vi "XXPathPlanner_Path_RePlan_Worker2.vi"(4 "StartingPoseTranslation":T11 {"Y" format="%14.3f"; "X" format="%14.3f"}, 5 "in PathPlannerPath":T1={"Reversed"=FALSE, "RotationTargets"=[], "ConstraintZones"=[], "EventMarkers"=[], "GlobalConstraints"={"MaxVelocityMps;"=0.0, "MaxAccelerationMpsSq;"=0.0, "MaxAngularVelRadPsEc;"=0.0, "MaxAngularAccRadPSecSq"=0.0, "Exists"=FALSE, "Unlimited"=FALSE, "NominalVoltageVolts"=12.0}, "GoalEndState"={"VelocityMPS"=0.0, "Rotation"={"VALUE"=0.0, "COS"=0.0, "SIN"=0.0}}, "AllPoints"=[], "Name"="", "Waypoints"=[], "PointTowardsZones"=[], "IdealStartingState"={"VelocityMPS"=0.0, "Rotation"={"VALUE"=0.0, "COS"=0.0, "SIN"=0.0}}, "IsChoreoPath"=FALSE, "PreventFlipping"=FALSE} {"IdealStartingState"."Rotation"."SIN" format="%13.4f"; "IdealStartingState"."Rotation"."COS" format="%13.4f"; "IdealStartingState"."Rotation"."VALUE" format="%13.4f"; "PointTowardsZones"."TargetPosition"."Y" format="%14.3f"; "PointTowardsZones"."TargetPosition"."X" format="%14.3f"; "PointTowardsZones"."RotationOffset"."SIN" format="%13.4f"; "PointTowardsZones"."RotationOffset"."COS" format="%13.4f"; "PointTowardsZones"."RotationOffset"."VALUE" format="%13.4f"; "Waypoints"."nextControl"."Y" format="%14.3f"; "Waypoints"."nextControl"."X" format="%14.3f"; "Waypoints"."anchor"."Y" format="%14.3f"; "Waypoints"."anchor"."X" format="%14.3f"; "Waypoints"."prevControl"."Y" format="%14.3f"; "Waypoints"."prevControl"."X" format="%14.3f"; "AllPoints"."RotationTarget"."rotation"."SIN" format="%13.4f"; "AllPoints"."RotationTarget"."rotation"."COS" format="%13.4f"; "AllPoints"."RotationTarget"."rotation"."VALUE" format="%13.4f"; "AllPoints"."Position"."Y" format="%14.3f"; "AllPoints"."Position"."X" format="%14.3f"; "GoalEndState"."Rotation"."SIN" format="%13.4f"; "GoalEndState"."Rotation"."COS" format="%13.4f"; "GoalEndState"."Rotation"."VALUE" format="%13.4f"; "RotationTargets"."rotation"."SIN" format="%13.4f"; "RotationTargets"."rotation"."COS" format="%13.4f"; "RotationTargets"."rotation"."VALUE" format="%13.4f"}) -> (2 "Error":bool, 3 "Replanned Path":T1={"Reversed"=FALSE, "RotationTargets"=[], "ConstraintZones"=[], "EventMarkers"=[], "GlobalConstraints"={"MaxVelocityMps;"=0.0, "MaxAccelerationMpsSq;"=0.0, "MaxAngularVelRadPsEc;"=0.0, "MaxAngularAccRadPSecSq"=0.0, "Exists"=FALSE, "Unlimited"=FALSE, "NominalVoltageVolts"=12.0}, "GoalEndState"={"VelocityMPS"=0.0, "Rotation"={"VALUE"=0.0, "COS"=0.0, "SIN"=0.0}}, "AllPoints"=[], "Name"="", "Waypoints"=[], "PointTowardsZones"=[], "IdealStartingState"={"VelocityMPS"=0.0, "Rotation"={"VALUE"=0.0, "COS"=0.0, "SIN"=0.0}}, "IsChoreoPath"=FALSE, "PreventFlipping"=FALSE} {"IdealStartingState"."Rotation"."SIN" format="%13.4f"; "IdealStartingState"."Rotation"."COS" format="%13.4f"; "IdealStartingState"."Rotation"."VALUE" format="%13.4f"; "PointTowardsZones"."TargetPosition"."Y" format="%14.3f"; "PointTowardsZones"."TargetPosition"."X" format="%14.3f"; "PointTowardsZones"."RotationOffset"."SIN" format="%13.4f"; "PointTowardsZones"."RotationOffset"."COS" format="%13.4f"; "PointTowardsZones"."RotationOffset"."VALUE" format="%13.4f"; "Waypoints"."nextControl"."Y" format="%14.3f"; "Waypoints"."nextControl"."X" format="%14.3f"; "Waypoints"."anchor"."Y" format="%14.3f"; "Waypoints"."anchor"."X" format="%14.3f"; "Waypoints"."prevControl"."Y" format="%14.3f"; "Waypoints"."prevControl"."X" format="%14.3f"; "AllPoints"."RotationTarget"."rotation"."SIN" format="%13.4f"; "AllPoints"."RotationTarget"."rotation"."COS" format="%13.4f"; "AllPoints"."RotationTarget"."rotation"."VALUE" format="%13.4f"; "AllPoints"."Position"."Y" format="%14.3f"; "AllPoints"."Position"."X" format="%14.3f"; "GoalEndState"."Rotation"."SIN" format="%13.4f"; "GoalEndState"."Rotation"."COS" format="%13.4f"; "GoalEndState"."Rotation"."VALUE" format="%13.4f"; "RotationTargets"."rotation"."SIN" format="%13.4f"; "RotationTargets"."rotation"."COS" format="%13.4f"; "RotationTargets"."rotation"."VALUE" format="%13.4f"})   [LabVIEW 2019]
doc: "Replan path worker 2\n\nInternal routine. Not for end user use."
uses:
  PathPlanner24.lvlib
  <vilib>/Rock Robotics/WPI/ThirdParty/JAS_Junk/TrajLib/Trajectory_Library.lvlib
  <vilib>/Rock Robotics/WPI/ThirdParty/JAS_Junk/TrajLib/TypeDef/TRANSLATION2D.ctl
  <vilib>/Rock Robotics/WPI/ThirdParty/JAS_Junk/TrajLib/TypeDef/ROTATION2D.ctl
  TypeDef/PathPlannerRotationTarget.ctl
  TypeDef/PathPlannerPathConstraints.ctl
  TypeDef/PathPlannerConstraintsZone.ctl
  ENum/PathPlanner_CommandUtilType_ENUM.ctl
  TypeDef/PathPlannerCommandUtil.ctl
  TypeDef/PathPlannerEventMarker.ctl
  TypeDef/PathPlannerGoalEndState.ctl
  TypeDef/PathPlannerPathPoint.ctl
  TypeDef/PathPlannerPath.ctl
  TypeDef/PathPlannerWaypoint.ctl
  TypeDef/PathPlannerPointTowardsZone.ctl
  TypeDef/PathPlannerIdealStartingState.ctl
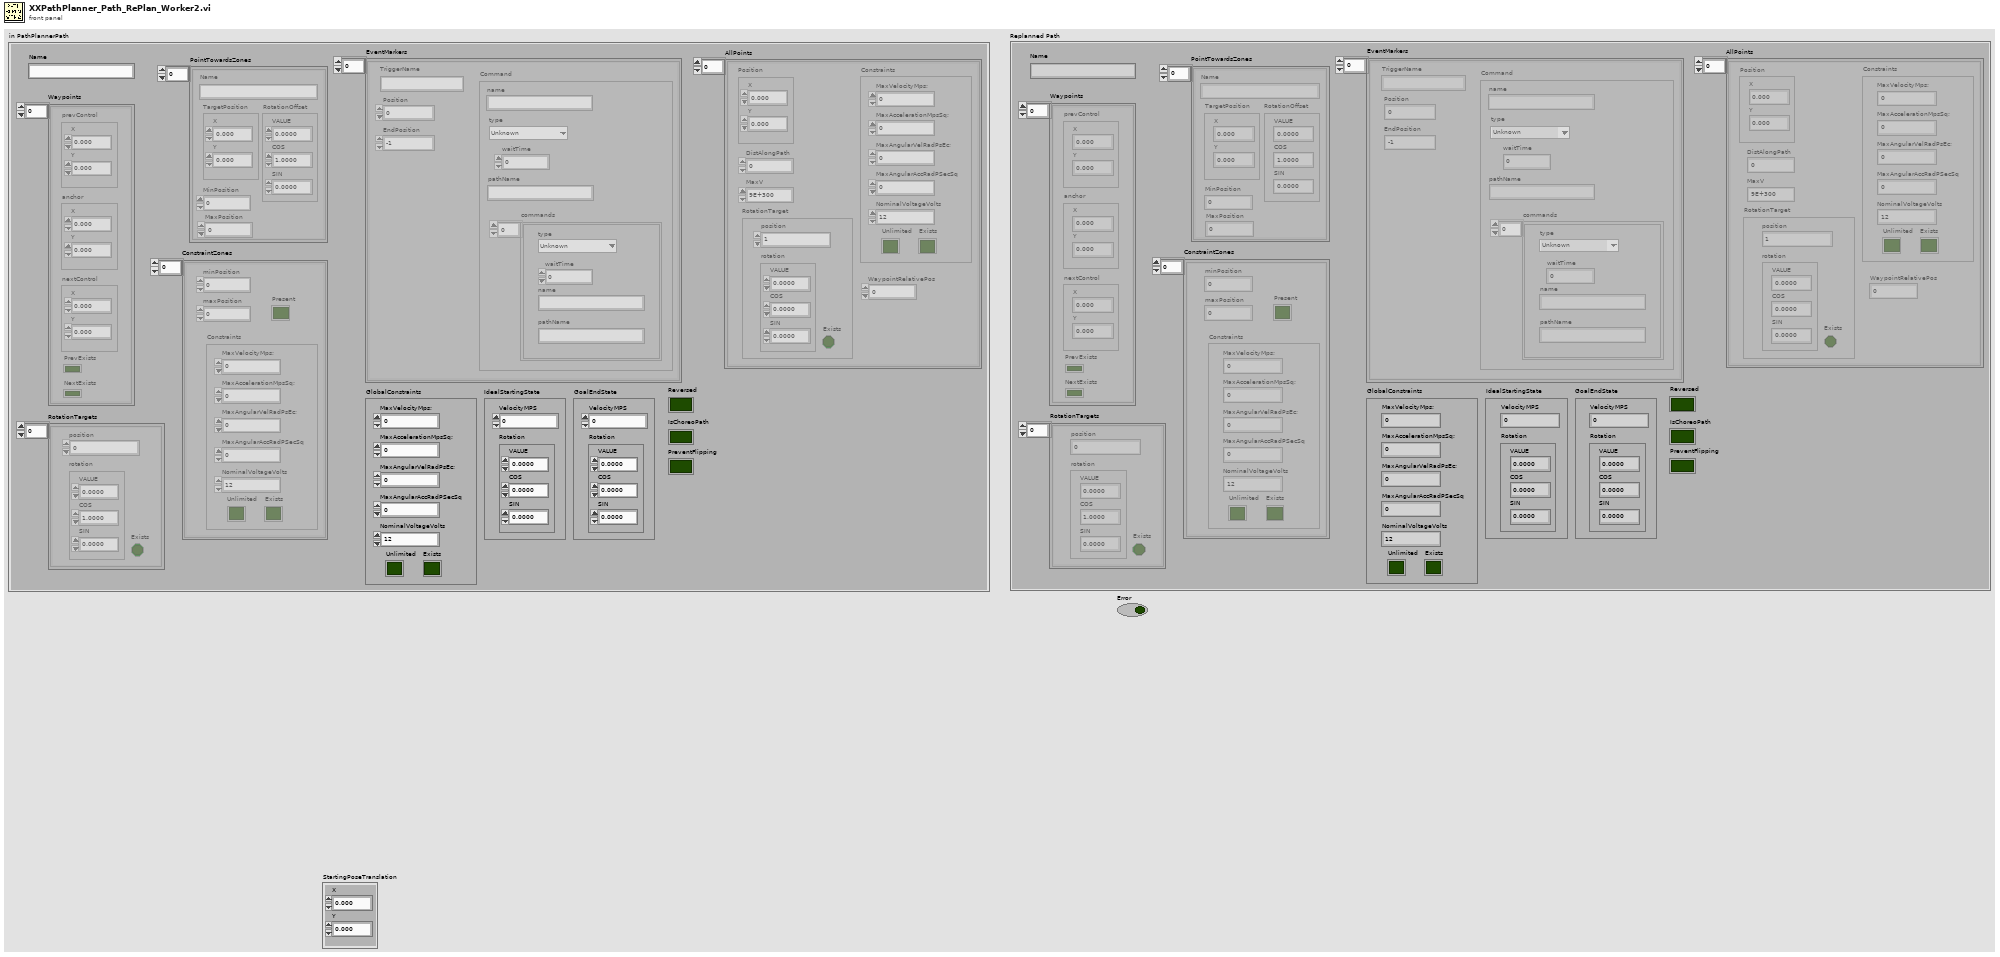
[diagram p1: front panel]
types:
  T1 = typedef "PathPlanner24.lvlib/PathPlannerPath.ctl" = cluster{"Reversed":bool, "RotationTargets":T2[], "ConstraintZones":T4[], "EventMarkers":T6[], "GlobalConstraints":T5, "GoalEndState":T9, "AllPoints":T10[], "Name":string, "Waypoints":T12[], "PointTowardsZones":T13[], "IdealStartingState":T14, "IsChoreoPath":bool, "PreventFlipping":bool}
  T2 = typedef "PathPlanner24.lvlib/PathPlannerRotationTarget.ctl" = cluster{"rotation":T3, "position":dbl, "Exists":bool}
  T3 = typedef "Trajectory_Library.lvlib/ROTATION2D.ctl" = cluster{"VALUE":dbl, "COS":dbl, "SIN":dbl}
  T4 = typedef "PathPlanner24.lvlib/PathPlannerConstraintsZone.ctl" = cluster{"minPosition":dbl, "maxPosition":dbl, "Constraints":T5, "Present":bool}
  T5 = typedef "PathPlanner24.lvlib/PathPlannerPathConstraints.ctl" = cluster{"MaxVelocityMps;":dbl, "MaxAccelerationMpsSq;":dbl, "MaxAngularVelRadPsEc;":dbl, "MaxAngularAccRadPSecSq":dbl, "Exists":bool, "Unlimited":bool, "NominalVoltageVolts":dbl}
  T6 = typedef "PathPlanner24.lvlib/PathPlannerEventMarker.ctl" = cluster{"Position":dbl, "Command":T7, "TriggerName":string, "EndPosition":dbl}
  T7 = typedef "PathPlanner24.lvlib/PathPlannerCommandUtil.ctl" = cluster{"waitTime":dbl, "name":string, "pathName":string, "commands":cluster{"type":T8, "waitTime":dbl, "name":string, "pathName":string}[], "type":T8}
  T8 = typedef "PathPlanner24.lvlib/PathPlanner_CommandUtilType_ENUM.ctl" = enum16{"Unknown", "Wait", "Named", "Path", "Sequential", "Parallel", "Race", "Deadline"}
  T9 = typedef "PathPlanner24.lvlib/PathPlannerGoalEndState.ctl" = cluster{"VelocityMPS":dbl, "Rotation":T3}
  T10 = typedef "PathPlanner24.lvlib/PathPlannerPathPoint.ctl" = cluster{"Position":T11, "DistAlongPath":dbl, "MaxV":dbl, "Constraints":T5, "RotationTarget":T2, "WaypointRelativePos":dbl}
  T11 = typedef "Trajectory_Library.lvlib/TRANSLATION2D.ctl" = cluster{"X":dbl, "Y":dbl}
  T12 = typedef "PathPlanner24.lvlib/PathPlannerWaypoint.ctl" = cluster{"prevControl":T11, "anchor":T11, "nextControl":T11, "PrevExists":bool, "NextExists":bool}
  T13 = typedef "PathPlanner24.lvlib/PathPlannerPointTowardsZone.ctl" = cluster{"RotationOffset":T3, "Name":string, "TargetPosition":T11, "MinPosition":dbl, "MaxPosition":dbl}
  T14 = typedef "PathPlanner24.lvlib/PathPlannerIdealStartingState.ctl" = cluster{"VelocityMPS":dbl, "Rotation":T3}
  T15 = typedef "PathPlannerPathSegment.ctl" = cluster{"SegmentPoints":T10[]}
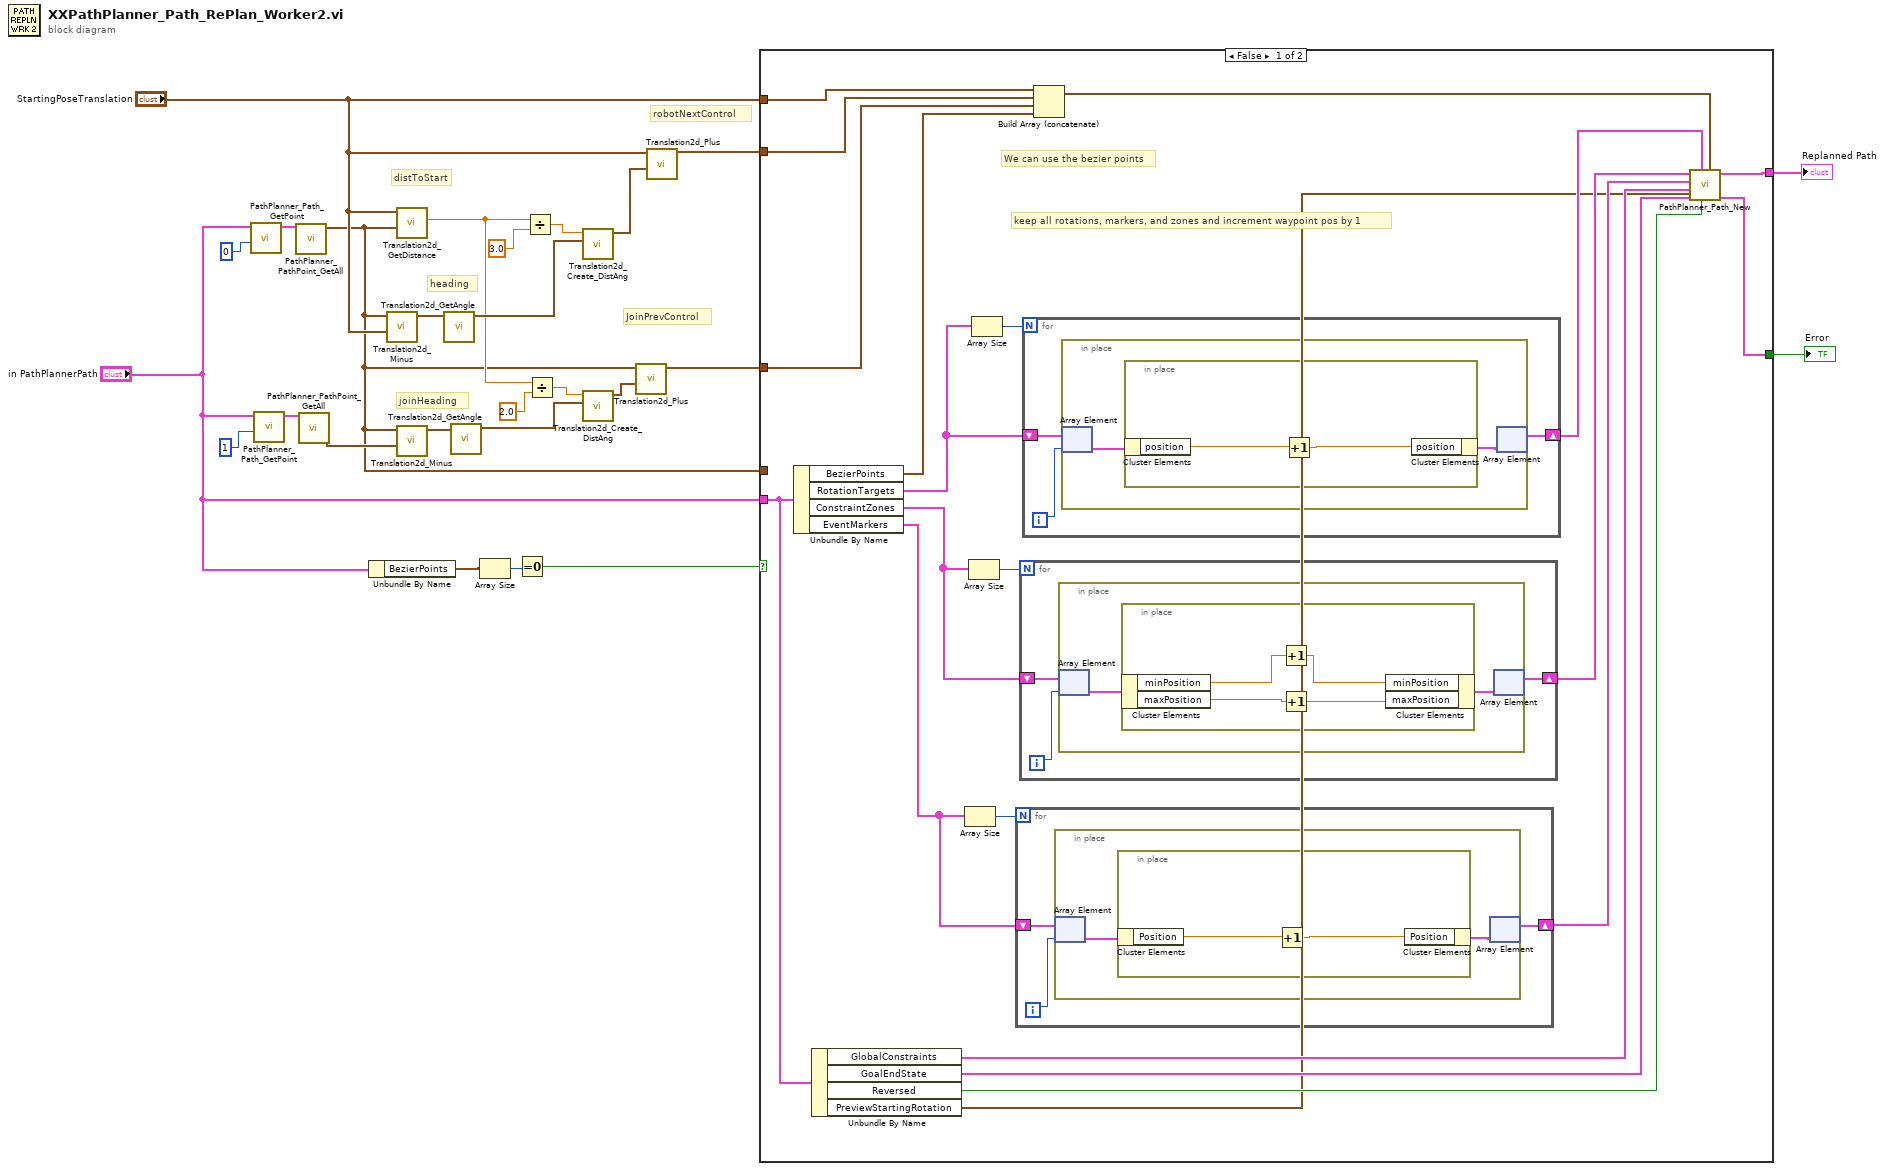
[diagram p0: block diagram]
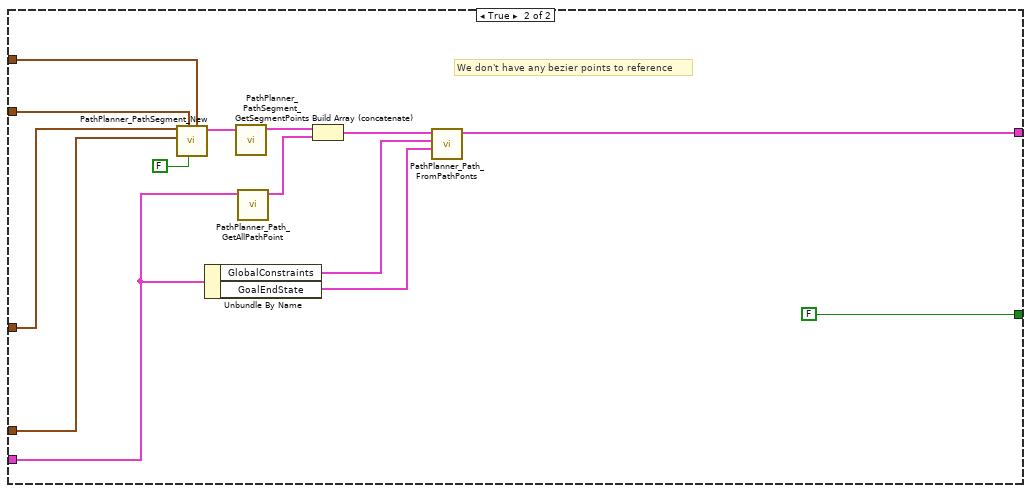
[diagram p2: hidden frame]
diagram:
  # "JoinPrevControl"
  # "joinHeading"
  # "robotNextControl"
  # "heading"
  # "distToStart"
  n1 = call "PathPlanner_Path_GetPoint.vi"("Index"=0, "PathPlannerPath"="in PathPlannerPath") -> ("Point"=w24:T10)  [unwired: 9 in]
  n2 = call "PathPlanner_Path_GetPoint.vi"("Index"=1, "PathPlannerPath"="in PathPlannerPath") -> ("Point"=w18:T10)  [unwired: 9 in]
  n3 = call "PathPlanner_PathPoint_GetAll.vi"("PathPlannerPoint"=w24) -> ("Position"=w5:T11)  [unwired: 5 in, 5 out]
  n4 = call "PathPlanner_PathPoint_GetAll.vi"("PathPlannerPoint"=w18) -> ("Position"=w17:T11)  [unwired: 5 in, 5 out]
  n5 = Unbundle By Name("in PathPlannerPath") -> ("BezierPoints"=w10:T11[])
  n6 = call <vilib>:"Translation2d_Minus.vi"("other Translation"="StartingPoseTranslation", "In Translation"=w5) -> ("Out Translation"=w26:T11)  [unwired: 9 in]
  n7 = call <vilib>:"Translation2d_GetDistance.vi"("other Translation"=w5, "In Translation"="StartingPoseTranslation") -> ("Distance"=w13:dbl)  [unwired: 9 in]
  n8 = call <vilib>:"Translation2d_Minus.vi"("other Translation"=w17, "In Translation"=w5) -> ("Out Translation"=w12:T11)  [unwired: 9 in]
  n9 = call <vilib>:"Translation2d_GetAngle.vi"("In Translation"=w26) -> ("Angle_Rotation2d"=w21:T3)  [unwired: 10 in]
  n10 = call <vilib>:"Translation2d_GetAngle.vi"("In Translation"=w12) -> ("Angle_Rotation2d"=w11:T3)  [unwired: 10 in]
  n11 = Array Size(array=w10) -> (size(s)=w9:i32)
  n12 = Equal To 0?(x=w9) -> (x = 0?=w8:bool)
  n13 = Divide(x=w13, y=3.0 ("Distance")) -> (x/y=w22:dbl)
  n14 = Divide(x=w13, y=2.0 ("Distance")) -> (x/y=w14:dbl)
  n15 = call <vilib>:"Translation2d_Create_DistAng.vi"("Angle"=w21, "Dist"=w22) -> ("TRANSLATION"=w20:T11)  [unwired: 9 in]
  n16 = call <vilib>:"Translation2d_Create_DistAng.vi"("Angle"=w11, "Dist"=w14) -> ("TRANSLATION"=w16:T11)  [unwired: 9 in]
  n17 = call <vilib>:"Translation2d_Plus.vi"("other Translation"=w16, "In Translation"=w5) -> ("Out Translation"=w6:T11)  [unwired: 9 in]
  n18 = call <vilib>:"Translation2d_Plus.vi"("other Translation"=w20, "In Translation"="StartingPoseTranslation") -> ("Out Translation"=w1:T11)  [unwired: 9 in]
  n19 = case shown="False" w8 {
    tunnel: "StartingPoseTranslation" -> [w41 w84]
    tunnel: w6 -> [w39 w82]
    tunnel: w5 -> [_ w81]
    tunnel: "in PathPlannerPath" -> [w31 w75]
    tunnel: [w37 w72] -> w3
    tunnel: [w36 FALSE] -> w2
    tunnel: w1 -> [w40 w83]
    frame False {
      # "keep all rotations, markers, and zones and increment waypoint pos by 1"
      # "We can use the bezier points"
      n20 = Unbundle By Name(w31) -> ("BezierPoints"=w38:T11[], "RotationTargets"=w46:T2[], "ConstraintZones"=w43:T4[], "EventMarkers"=w42:T6[])
      n21 = Unbundle By Name(w31) -> ("GlobalConstraints"=w30:T5, "GoalEndState"=w29:T9, "Reversed"=w28:bool, "PreviewStartingRotation"=w27:T3)
      n22 = Array Size(array=w42) -> (size(s)=w44:i32)
      n23 = Array Size(array=w43) -> (size(s)=w45:i32)
      n24 = Array Size(array=w46) -> (size(s)=w47:i32)
      n25 = for {
        N: w44 -> [_]
        shift-right: [w48] -> w32
        shift-left: w42 -> [w49]
        i -> [w50]
        n26 = in-place {
          n27 = in-place-array #1(w49, w50) -> (w52:T6)
          n28 = in-place {
            n29 = in-place-cluster #2(w52) -> ("Position"=w54:dbl)
            n30 = Increment(x=w54) -> (x+1=w53:dbl)
            n31 = in-place-cluster #2("Position"=w53) -> (w51:T6)
          }
          n32 = in-place-array #1(w51) -> (w48:T6[])  [unwired: 1 out]
        }
      }
      n33 = for {
        N: w45 -> [_]
        shift-right: [w55] -> w33
        shift-left: w43 -> [w56]
        i -> [w57]
        n34 = in-place {
          n35 = in-place-array #3(w56, w57) -> (w59:T4)
          n36 = in-place {
            n37 = in-place-cluster #4(w59) -> ("minPosition"=w63:dbl, "maxPosition"=w61:dbl)
            n38 = Increment(x=w63) -> (x+1=w62:dbl)
            n39 = Increment(x=w61) -> (x+1=w60:dbl)
            n40 = in-place-cluster #4("minPosition"=w62, "maxPosition"=w60) -> (w58:T4)
          }
          n41 = in-place-array #3(w58) -> (w55:T4[])  [unwired: 1 out]
        }
      }
      n42 = for {
        N: w47 -> [_]
        shift-right: [w64] -> w34
        shift-left: w46 -> [w65]
        i -> [w66]
        n43 = in-place {
          n44 = in-place-array #5(w65, w66) -> (w68:T2)
          n45 = in-place {
            n46 = in-place-cluster #6(w68) -> ("position"=w70:dbl)
            n47 = Increment(x=w70) -> (x+1=w69:dbl)
            n48 = in-place-cluster #6("position"=w69) -> (w67:T2)
          }
          n49 = in-place-array #5(w67) -> (w64:T2[])  [unwired: 1 out]
        }
      }
      n50 = Build Array (concatenate)(w41, w40, w39, w38) -> (w35:T11[])
      n51 = call "PathPlanner_Path_New.vi"("IdealStartingState"=w27, "Waypoints"=w35, "Reversed"=w28, "HolonomicRotations"=w34, "GoalEndState"=w29, "GlobalConstraints"=w30, "EventMarkers"=w32, "ConstraintZones"=w33) -> ("PointTowardsZones"=w36:T13[], "PathPlannerPath"=w37:T1)  [unwired: 1 in, 1 out]
    }
    frame True {
      # "We don't have any bezier points to reference"
      n52 = call "PathPlanner_PathSegment_New.vi"("P1"=w84, "EndSegment"=FALSE, "P2"=w83, "P4"=w81, "P3"=w82) -> ("Segment"=w79:T15)  [unwired: 6 in]
      n53 = Unbundle By Name(w75) -> ("GlobalConstraints"=w74:T5, "GoalEndState"=w73:T9)
      n54 = call "PathPlanner_PathSegment_GetSegmentPoints.vi"("Segment"=w79) -> ("SegmentPoints"=w78:T10[])  [unwired: 10 in]
      n55 = call "PathPlanner_Path_GetAllPathPoint.vi"("PathPlannerPath"=w75) -> ("AllPoints"=w77:T10[])  [unwired: 10 in]
      n56 = Build Array (concatenate)(w78, w77) -> (w76:T10[])
      n57 = call "PathPlanner_Path_FromPathPonts.vi"("GoalEndState"=w73, "GlobalConstraints"=w74, "PathPoints"=w76) -> ("PathPlannerPath"=w72:T1)  [unwired: 8 in]
    }
  }
  "Error" <- w2
  "Replanned Path" <- w3
